vi "xiLIB - ErrorHandler_UNUSED.vi"(8 "error in (no error)":errorcluster) -> (0 "error out":errorcluster)   [LabVIEW 2013]
doc: "Returns the current GPI States of Currera Camera."
uses:
  Globals/xiLIB - PRM_Info.vi
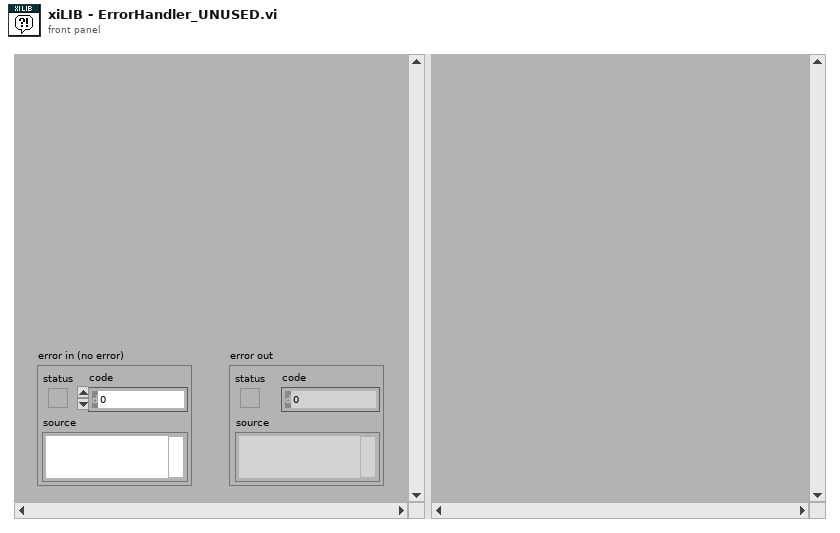
[diagram p1: front panel]
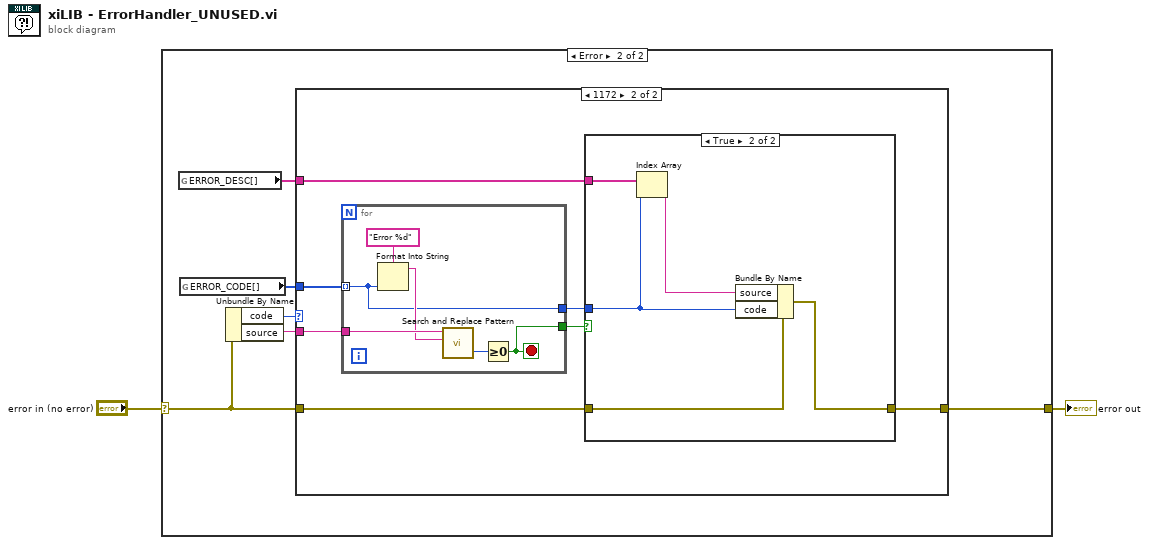
[diagram p0: block diagram]
diagram:
  n1 = case shown="Error" "error in (no error)" {
    selector: "error in (no error)" -> [w3 w8]
    tunnel: [w3 w7] -> w1
    frame No Error {
    }
    frame Error {
      n2 = global read "xiLIB - PRM_Info.vi" "ERROR_DESC[]"() -> (w4:string[])
      n3 = global read "xiLIB - PRM_Info.vi" "ERROR_CODE[]"() -> (w5:i32[])
      n4 = Unbundle By Name(w8) -> ("code"=w9:i32, "source"=w6:string)
      n5 = case shown="1172" w9 {
        tunnel: w8 -> [w10 w14]
        tunnel: [w10 w11] -> w7
        tunnel: w6 -> [_ w16]
        tunnel: w5 -> [_ w17]
        tunnel: w4 -> [_ w12]
        frame Default {
        }
        frame 1172 {
          n6 = for {
            tunnel: w17 -> [w24] mode=indexing
            tunnel: w16 -> [w28]
            tunnel: [w25] -> w15
            tunnel: [w24] -> w13
            stop <- w25 stop-if-true
            n7 = Format Into String(format string="Error %d", w24) -> (resulting string=w27:string)  [unwired: 2 in, 1 out]
            n8 = call <vilib>:"Search and Replace Pattern.vi"("string"=w28, "regular expression (\"\")"=w27) -> ("offset past match"=w26:i32)  [unwired: 3 in, 1 out]
            n9 = Greater Or Equal To 0?(x=w26) -> (x >= 0?=w25:bool)
          }
          n10 = case shown="True" w15 {
            tunnel: w14 -> [w18 w23]
            tunnel: w13 -> [_ w21]
            tunnel: w12 -> [_ w22]
            tunnel: [w18 w19] -> w11
            frame False {
            }
            frame True {
              n11 = Index Array(array=w22, index=w21) -> (element=w20:string)
              n12 = Bundle By Name(cluster=w23, "source"=w20, "code"=w21) -> (w19:errorcluster)
            }
          }
        }
      }
    }
  }
  "error out" <- w1
